vi "drift corrected gate current sweep.vi"() -> ()   [LabVIEW 2010]
uses:
  <vilib>/Utility/file.llb/Write To Spreadsheet File (DBL).vi
  <userlib>/Nanonis Prog Interface V5/Nanonis Prog Interface.lvlib
panel:
  out "Index":i32
  out "XY Graph":cluster{dbl[], sgl[]}(graph)
  in  "Number of Z Averages":i32=1
  in  "Number of Current Averages":i32=20
  out "Current Gate Voltage (V)":dbl
  in  "Increment Gate (V)":dbl
  in  "End Gate (V)":dbl
  in  "Start Gate (V)":dbl
  in  "Filename":string
  # "DRIFT CORRECTED\nGate-Current Sweep"
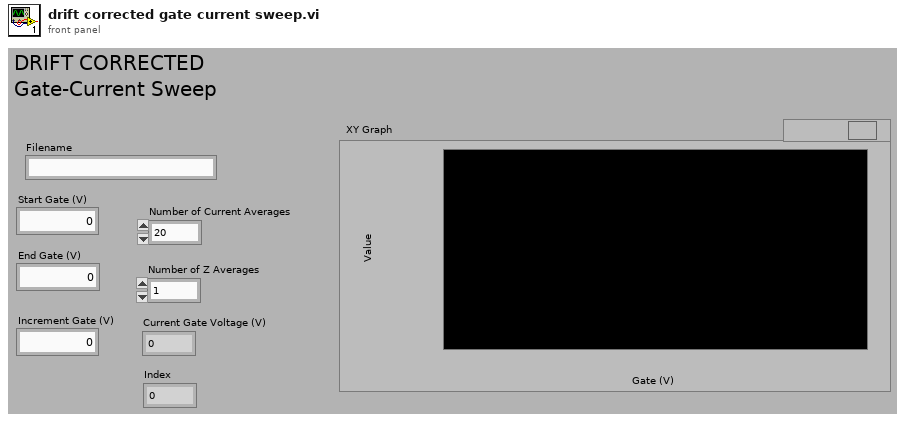
[diagram p1: front panel]
types:
  T1 = enum16{"Set Voltage", "Read Voltage", "Read Setpoint", "Read Current", "Output On", "Output Off"}
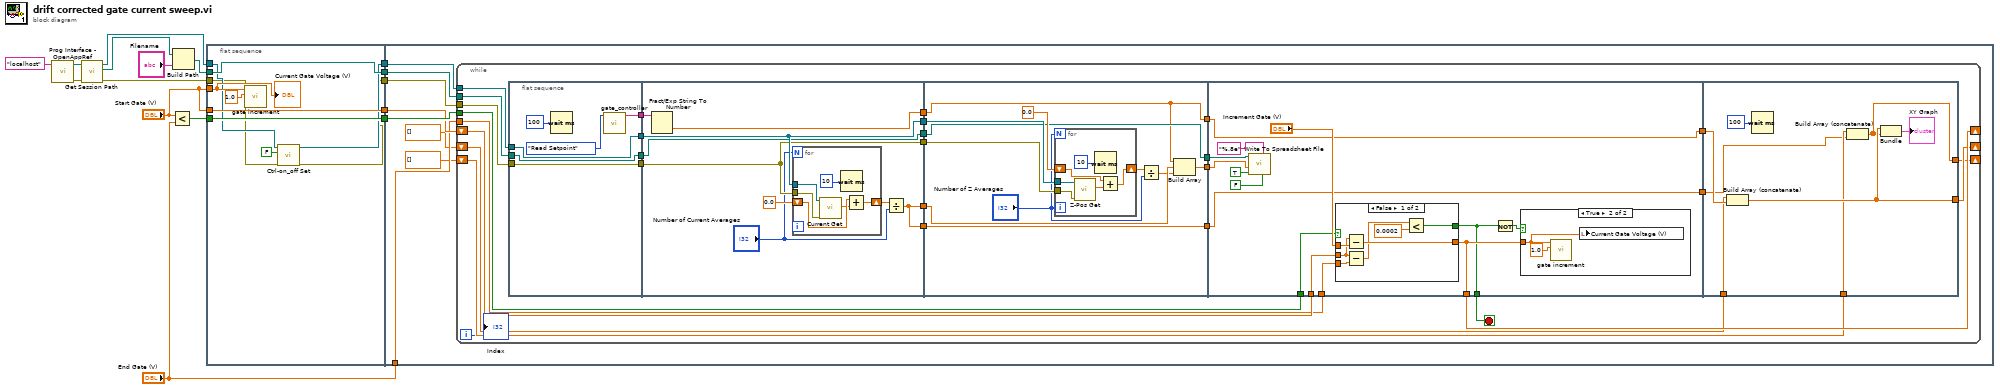
[diagram p0: block diagram]
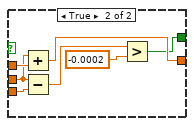
[diagram p2: hidden frame]
diagram:
  n1 = call <userlib>:"Prog Interface - OpenAppRef.vi"("Machine name (local machine IP)"="localhost" ("machine name (localhost)")) -> ("Error out"=w8:errorcluster, "Application reference"=w9:refnum<vi>)  [unwired: 5 in]
  n2 = call <userlib>:"Get Session Path.vi"("error in (no error)"=w8, "Application ref in"=w9) -> ("error out"=w7:errorcluster, "Session path"=w5:path, "Application ref out"=w6:refnum<vi>)  [unwired: 7 in]
  n3 = Less?(x="Start Gate (V)", y="End Gate (V)") -> (x < y?=w15:bool)
  n4 = Build Path(base path=w5, name or relative path="Filename") -> (appended path=w3:path)
  n5 = flat-sequence {
    tunnel: "Start Gate (V)" -> [w25]
    tunnel: w15 -> [w26]
    tunnel: w6 -> [w19]
    tunnel: w7 -> [w18]
    tunnel: [w17] -> w14
    tunnel: [w26] -> w13
    tunnel: [w25] -> w12
    tunnel: "Start Gate (V)" -> [w23]
    tunnel: w3 -> [w22]
    tunnel: [w22] -> w2
    tunnel: [w20] -> w1
    tunnel: w14 -> [w34]
    tunnel: w13 -> [w32]
    tunnel: w12 -> [w31]
    tunnel: "End Gate (V)" -> [w30]
    tunnel: w2 -> [w29]
    tunnel: w1 -> [w33]
    frame #0 {
      n6 = call "gate increment.vi"("Increment"=1.0, "Gate Voltage"=w23) -> ()  [unwired: 10 in]
      n7 = call <userlib>:"Ctrl-on_off Set.vi"("error in (no error)"=w18, "Z Controller ON/OFF"=FALSE, "Application ref in"=w19) -> ("error out"=w17:errorcluster, "Application ref out"=w20:refnum<vi>)  [unwired: 7 in]
      "Current Gate Voltage (V)" <- w23
    }
    frame #1 {
      n8 = while {
        tunnel: w34 -> [w63]
        tunnel: w33 -> [w62]
        tunnel: w32 -> [w56]
        shift-right: [w59] -> _
        shift-left: w31 -> [w58]
        tunnel: w30 -> [w57]
        tunnel: w29 -> [w48]
        shift-right: [w42] -> _
        shift-left: dbl[] [] -> [w41]
        shift-right: [w37] -> _
        shift-left: sgl[] [] -> [w36]
        i -> [w35]
        stop <- w55 stop-if-true
        n9 = flat-sequence {
          tunnel: w62 -> [w68]
          tunnel: w63 -> [w69]
          tunnel: [w69] -> w61
          tunnel: [w68] -> w60
          tunnel: [w65] -> w52
          tunnel: w48 -> [w64]
          tunnel: [w64] -> w45
          tunnel: w61 -> [w76]
          tunnel: w60 -> [w77]
          tunnel: [w77] -> w54
          tunnel: [w76] -> w53
          tunnel: w52 -> [w73]
          tunnel: [w72] -> w51
          tunnel: [w70] -> w50
          tunnel: [w71] -> w46
          tunnel: w45 -> [w71]
          tunnel: [w70] -> w38
          tunnel: w54 -> [w94]
          tunnel: w53 -> [w93]
          tunnel: w51 -> [w87]
          tunnel: w50 -> [w90]
          tunnel: [w89] -> w49
          tunnel: [w88] -> w47
          tunnel: w46 -> [w88]
          tunnel: [w87] -> w44
          tunnel: [w86] -> w39
          tunnel: w38 -> [w86]
          tunnel: [w115] -> w59
          tunnel: [w114] -> w55
          tunnel: w58 -> [w113]
          tunnel: w57 -> [w111]
          tunnel: w56 -> [w110]
          tunnel: w49 -> [w106]
          tunnel: w47 -> [w105]
          tunnel: w44 -> [w103]
          tunnel: [w103] -> w43
          tunnel: [w102] -> w40
          tunnel: w39 -> [w102]
          tunnel: w43 -> [w137]
          tunnel: [w136] -> w42
          tunnel: w41 -> [w135]
          tunnel: w40 -> [w132]
          tunnel: [w134] -> w37
          tunnel: w36 -> [w133]
          frame #0 {
            n10 = Wait (ms)(milliseconds to wait=u32 100) -> ()  [unwired: 1 out]
            n11 = call "gate_controller.vi"("Command"=T1."Read Setpoint") -> ("Response"=w65:string)  [unwired: 10 in]
          }
          frame #1 {
            n12 = Fract/Exp String To Number(string=w73) -> (number=w72:dbl)  [unwired: 3 in, 1 out]
            n13 = for {
              N: "Number of Current Averages" -> [_]
              tunnel: w77 -> [w84]
              tunnel: w76 -> [w83]
              shift-right: [w82] -> w75
              shift-left: sgl 0.0 ("Current (A)") -> [w81]
              n14 = call <userlib>:"Current Get.vi"("Error in (no error)"=w83, "Application ref in"=w84) -> ("Current (A)"=w80:sgl)  [unwired: 5 in, 2 out]
              n15 = Wait (ms)(milliseconds to wait=u32 10) -> ()  [unwired: 1 out]
              n16 = Add(x=w81, y=w80) -> (x+y=w82:sgl)
            }
            n17 = Divide(x=w75, y="Number of Current Averages") -> (x/y=w70:sgl)
          }
          frame #2 {
            n18 = for {
              N: "Number of Z Averages" -> [_]
              tunnel: w94 -> [w98]
              tunnel: w93 -> [w99]
              shift-right: [w101] -> w92
              shift-left: sgl 0.0 ("Current (A)") -> [w100]
              n19 = call <userlib>:"Z-Pos Get.vi"("error in (no error)"=w99, "Application ref in"=w98) -> ("Z position (m)"=w97:sgl)  [unwired: 7 in, 2 out]
              n20 = Wait (ms)(milliseconds to wait=u32 10) -> ()  [unwired: 1 out]
              n21 = Add(x=w100, y=w97) -> (x+y=w101:sgl)
            }
            n22 = Divide(x=w92, y="Number of Z Averages") -> (x/y=w85:sgl)
            n23 = Build Array(w87, w90, w85) -> (w89:dbl[])
          }
          frame #3 {
            n24 = call-poly <vilib>:"Write To Spreadsheet File.vi"("transpose? (no:F)"=FALSE, "format (%.3f)"="%.8e", "append to file? (new file:F)"=TRUE, "1D data"=w106, "file path (dialog if empty)"=w105) -> ()  [unwired: 3 in, 1 out]
            n25 = case shown="False" w110 {
              tunnel: w113 -> [w120 w126]
              tunnel: "Increment Gate (V)" -> [w121 w129]
              tunnel: [w122 w128] -> w115
              tunnel: w111 -> [w119 w127]
              tunnel: [w117 w125] -> w114
              frame False {
                n26 = Subtract(x=w120, y=w121) -> (x-y=w122:dbl)
                n27 = Subtract(x=w120, y=w119) -> (x-y=w118:dbl)
                n28 = Less?(x=w118, y=0.0002) -> (x < y?=w117:bool)
              }
              frame True {
                n29 = Add(x=w126, y=w129) -> (x+y=w128:dbl)
                n30 = Subtract(x=w126, y=w127) -> (x-y=w124:dbl)
                n31 = Greater?(x=w124, y=-0.0002) -> (0:w125:bool)
              }
            }
            n32 = Not(x=w114) -> (.not. x?=w109:bool)
            n33 = case shown="True" w109 {
              tunnel: w115 -> [_ w131]
              frame False {
              }
              frame True {
                n34 = call "gate increment.vi"("Increment"=1.0, "Gate Voltage"=w131) -> ()  [unwired: 10 in]
                n35 = local write "Current Gate Voltage (V)"(w131) -> ()
              }
            }
          }
          frame #4 {
            n36 = Build Array (concatenate)(w135, w137) -> (w136:dbl[])
            n37 = Wait (ms)(milliseconds to wait=u32 100) -> ()  [unwired: 1 out]
            n38 = Build Array (concatenate)(w133, w132) -> (w134:sgl[])
            n39 = Bundle(w136, w134) -> (→"XY Graph":cluster{dbl[], sgl[]})  [unwired: 1 in]
          }
        }
        "Index" <- w35
      }
    }
  }
